vi "Drivetrain Yaw Rate Compensation.vi"(10 "Steer in":dbl) -> (1 "Yaw Comp Indicators":T1, 2 "Steer Out":dbl)   [LabVIEW 2014]
uses:
  Common Code/Yaw Rate Compensation Indicators.ctl
  Robot Global Data.vi
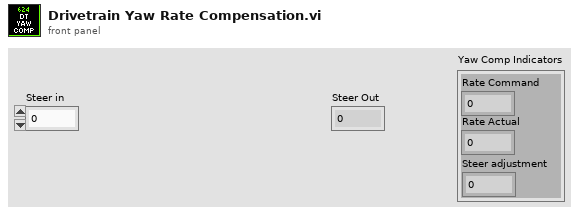
[diagram p1: front panel]
types:
  T1 = typedef "Yaw Rate Compensation Indicators.ctl" = cluster{"Rate Command":sgl, "Rate Actual":sgl, "Steer adjustment":sgl}
  T2 = typedef "Dashboard Control Data.ctl" = cluster{"Cam Exposure":dbl, "Go to angle":dbl, "Steer PID Gains":cluster{"proportional gain (Kc)":dbl, "integral time (Ti, min)":dbl, "derivative time (Td, min)":dbl}, "Steer PID output Range":cluster{"output high":dbl, "output low":dbl}, "Pressure m \nValue":dbl, "Pressure b \nValue":dbl, "Roller Command Cluster ":T3, "Elevator":T4, "Encoder Control":T6, "Auton Settings":cluster{"Drive Dist Window Size":dbl}, "Drivetrain Settings":T7}
  T3 = typedef "Roller Control.ctl" = cluster{"Intake Speed":dbl, "Turn In Speed":dbl, "Unload Speed":dbl, "Turn Out Speed":dbl, "Ping Align Tolerance":dbl, "Tote Range Threshold":dbl, "Right Pot 0":dbl, "Pot Threshold":dbl, "Left Pot 0":dbl, "Manual 0s?":bool, "Right Pot Scale":dbl, "Left Pot Scale":dbl, "0 wait time":i32, "Zero Pots":bool, "Min Elevator Height":dbl, "Eject Time":dbl, "Eject US Threshold":dbl, "Anti-Twitch Time":u32, "Ping Caring Threshold":dbl, "Pot Diff Threshold":dbl, "Pinch Sustain":u32, "Absorb Give Up Threshold":dbl, "Untip In Threshold":dbl, "Untip Grab Range":dbl, "Ultrasonic Hold Time":u32, "Landscape Absorb Time":u32, "Pot Use Wait Time":u32, "Can Turn Stop Range":dbl}
  T4 = typedef "Elevator DB Control.ctl" = cluster{"PID Output Range":cluster{"output high":dbl, "output low":dbl}, "PID gains":cluster{"proportional gain (Kc)":dbl, "integral time (Ti, min)":dbl, "derivative time (Td, min)":dbl}, "Height Tolerance":sgl, " Encoder Constant":dbl, "Safe Mode Max Speed":sgl, "Eject Time":sgl, "Zeroing Speed":sgl, "Presets":T5, "Ping Detect Threshold":sgl, "Trashcan Detect Threshold":sgl, "Zero Filter Time":dbl, "Stabilizer Open Time":dbl, "Zero Creep Speed":dbl, "Max Current":dbl, "Current Trip Time":dbl, "Abort Pitch":dbl}
  T5 = typedef "Elevator Presets.ctl" = cluster{"Pickup 2 w/ Tote":sgl, "Pickup 2 w/ Trashcan":sgl, "Pickup 3 w/ Tote":sgl, "Pickup 3 w/ Trashcan":sgl, "Bottom":sgl, "Pickup 1 w/ Tote":sgl, "Pickup Trashcan":sgl, "Pickup 1 w/ Trashcan":sgl, "Eject":sgl, "Hold Low":sgl, "Step add height":sgl, "Store Trashcan 1":sgl, "Store Trashcan 2":sgl, "Store Trashcan 3":sgl, "6 Tote Max":sgl, "5 Tote Max":sgl, "Untip Lift":dbl, "Drop Stack":dbl, "Pickup 1 Empty":dbl, "Pickup 2 Empty":dbl, "Pickup 3 Empty":dbl, "4 Tote Max":dbl, "HP Load Hold":dbl, "HP Load Drop":dbl, "HP Load Finger":dbl, "HP Load Hold Can":dbl}
  T6 = typedef "Encoder Control.ctl" = cluster{"Left Tick Constant":dbl, "Right Tick Constant":dbl, "Center Tick Constant":dbl, "Reset?":bool, "Y Dist":cluster{"PID gains":cluster{"proportional gain (Kc)":dbl, "integral time (Ti, min)":dbl, "derivative time (Td, min)":dbl}}, "X Dist":cluster{"PID gains":cluster{"proportional gain (Kc)":dbl, "integral time (Ti, min)":dbl, "derivative time (Td, min)":dbl}}, "Y Stop Thresh":dbl, "Y Stop Speed":dbl, "X Stop Thresh":dbl, "X Stop Speed":dbl}
  T7 = typedef "Drivetrain Settings.ctl" = cluster{"Gyro Tolerance":dbl, "Strafe Correct max steer":dbl, "Strafe Timer Wait":dbl, "Throttle Ramp (ms)":dbl, "Strafe Ramp (ms)":dbl, "Angular rate compensation":bool, "Throttle to Rate Scale":dbl, "Rate compensation gain":dbl}
  T8 = typedef "IMU Data.ctl" = cluster{"Pitch":sgl, "Roll":sgl, "Yaw":sgl, "Data Valid?":bool, "Temp":sgl, "MOVING":bool, "NAVX_CAL_STATUS":T9, "NAVX_OP_STATUS":T10, "YAW_STABLE":bool, "Accel X":sgl, "Accel Y":sgl, "Accel Z":sgl, "Accel Magnitude":sgl, "Pitch Rate":sgl, "Roll Rate":sgl, "Yaw Rate":sgl}
  T9 = typedef "navX-MXP IMU.lvlib/navX NAVX_CAL_STATUS.ctl" = u8
  T10 = typedef "navX-MXP IMU.lvlib/navX NAVX_OP_STATUS.ctl" = u8
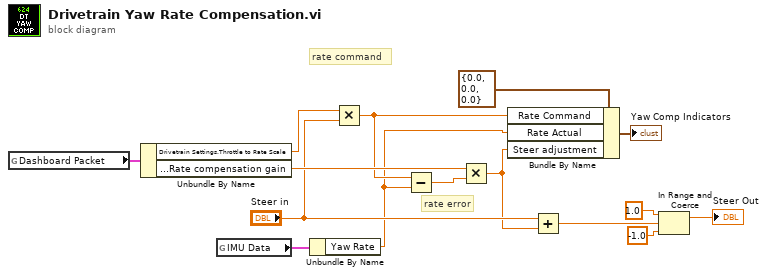
[diagram p0: block diagram]
diagram:
  # "rate error"
  # "rate command"
  n1 = global read "Robot Global Data.vi" "Dashboard Packet"() -> (w15:T2)
  n2 = Unbundle By Name(w15) -> ("Drivetrain Settings.Throttle to Rate Scale"=w14:dbl, "Drivetrain Settings.Rate compensation gain"=w11:dbl)
  n3 = global read "Robot Global Data.vi" "IMU Data"() -> (w13:T8)
  n4 = Unbundle By Name(w13) -> ("Yaw Rate"=w3:sgl)
  n5 = Multiply(x=w14, y="Steer in") -> (x*y=w4:dbl)
  n6 = Subtract(x=w4, y=w3) -> (x-y=w12:dbl)
  n7 = Multiply(x=w11, y=w12) -> (x*y=w2:dbl)
  n8 = Bundle By Name(cluster=T1 {"Rate Command"=0.0, "Rate Actual"=0.0, "Steer adjustment"=0.0} ("Yaw Comp Indicators"), "Rate Command"=w4, "Rate Actual"=w3, "Steer adjustment"=w2) -> (→"Yaw Comp Indicators":T1)
  n9 = Add(x="Steer in", y=w2) -> (x+y=w10:dbl)
  n10 = In Range and Coerce(upper limit=1.0, x=w10, lower limit=-1.0) -> (coerced(x)=→"Steer Out":dbl)  [unwired: 1 out]
